vi "MoveToPositionXYZ.vi"(11 "Array":dbl[](array[numeric])) -> ()   [LabVIEW 2020]
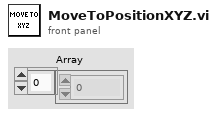
[diagram p1: front panel]
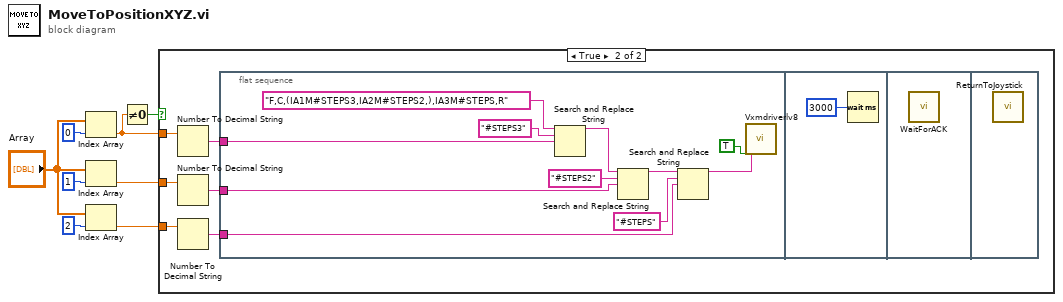
[diagram p0: block diagram]
diagram:
  n1 = Index Array(array="Array", index=0) -> (element=w2:dbl)
  n2 = Index Array(array="Array", index=1) -> (element=w4:dbl)
  n3 = Index Array(array="Array", index=2) -> (element=w3:dbl)
  n4 = Not Equal To 0?(x=w2) -> (x != 0?=w1:bool)
  n5 = case shown="True" w1 {
    tunnel: w4 -> [_ w12]
    tunnel: w3 -> [_ w11]
    tunnel: w2 -> [_ w9]
    frame False {
    }
    frame True {
      n6 = Number To Decimal String(number=w9) -> (decimal integer string=w14:string)  [unwired: 1 in]
      n7 = Number To Decimal String(number=w12) -> (decimal integer string=w13:string)  [unwired: 1 in]
      n8 = Number To Decimal String(number=w11) -> (decimal integer string=w10:string)  [unwired: 1 in]
      n9 = flat-sequence {
        tunnel: w13 -> [w20]
        tunnel: w14 -> [w19]
        tunnel: w10 -> [w16]
        frame #0 {
          n10 = Search and Replace String(input string="F,C,(IA1M#STEPS3,IA2M#STEPS2,),IA3M#STEPS,R" ("Chars to send"), search string="#STEPS3", replace string=w19) -> (result string=w23:string)  [unwired: 5 in, 3 out]
          n11 = Search and Replace String(input string=w23, search string="#STEPS2", replace string=w20) -> (result string=w15:string)  [unwired: 5 in, 3 out]
          n12 = Search and Replace String(input string=w15, search string="#STEPS", replace string=w16) -> (result string=w17:string)  [unwired: 5 in, 3 out]
          n13 = call "Vxmdriverlv8.Vi"("Send\nchars\nto port"=TRUE, "Chars to send"=w17) -> ()  [unwired: 20 in, 6 out]
        }
        frame #1 {
          n14 = Wait (ms)(milliseconds to wait=u32 3000) -> ()  [unwired: 1 out]
        }
        frame #2 {
          n15 = call "WaitForACK.vi"() -> ()  [unwired: 12 in]
        }
        frame #3 {
          n16 = call "ReturnToJoystick.vi"() -> ()  [unwired: 12 in]
        }
      }
    }
  }
